vi "EncodeFloat.vi"(1 "Data In":fxp<+/-,32,16>[](array[numeric]) format="%.4g") -> (0 "Data Out":u8[](array[numeric]))   [LabVIEW 2014, in "navX Library v1 (deprecated).lvlib"]
uses:
  navX Library v1 (deprecated).lvlib
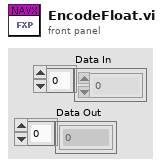
[diagram p1: front panel]
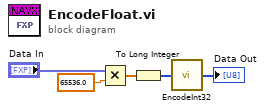
[diagram p0: block diagram]
diagram:
  n1 = Multiply(x="Data In", y=65536.0) -> (x*y=w4:dbl[])
  n2 = To Long Integer(number=w4) -> (32bit integer=w3:i32[])
  n3 = call "EncodeInt32.vi"("Data In"=w3) -> ("Data Out"=→"Data Out":u8[])
